vi "Periodic Tasks.vi"(8 "error in":errorcluster) -> ()   [LabVIEW 2019]
doc: "This VI runs in parallel to other tasks. It can contain as many user-defined periodic loops as you need. These can carry out PID or other sorts of timed response."
uses:
  <vilib>/Rock Robotics/WPI/Utilities/WPI_GetSetVariantRefNum.vi
  <vilib>/Rock Robotics/Network Tables/NT Read Boolean.vi
  <vilib>/Rock Robotics/Network Tables/NT Read Number.vi
  <vilib>/Rock Robotics/WPI/RobotDrive/WPI_RobotDriveArcadeDrive_Standard(NoSaturation).vi
  <vilib>/Rock Robotics/Network Tables/NT Write Numeric Array.vi
  <vilib>/Rock Robotics/Network Tables/NT Write Boolean.vi
  <vilib>/Rock Robotics/Network Tables/NT Write Number.vi
  <vilib>/Rock Robotics/Network Tables/NT Write String.vi
  <vilib>/Rock Robotics/Network Tables/NT Read String.vi
panel:
  out "Motor velocities":dbl[](array[knob]) scale=0.0..10.0
  out "Motor temperatures":dbl[](array[slide]) scale=100.0..250.0
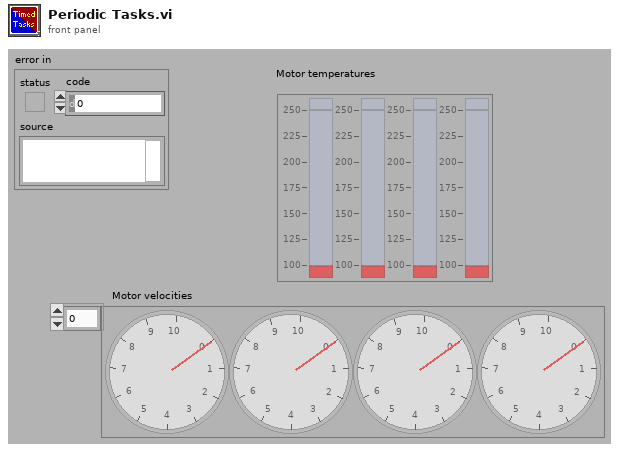
[diagram p1: front panel]
types:
  T1 = typedef "WPI_JoystickDevRef.ctl" = cluster{"Device":T2}
  T2 = typedef "WPI_JoystickDeviceEnum.ctl" = enum16{"USB 0", "USB 1", "USB 2", "USB 3", "USB 4", "USB 5"}
  T3 = typedef "WPI_RobotDriveDevRef.ctl" = cluster{"DevStatus":errorcluster, "Motors[]":T4[], "Square Inputs":bool, "Max Output":dbl}
  T4 = typedef "WPI_MotorControlDeviceRef.ctl" = cluster{"DeviceStatus":errorcluster, "Type":T5, "PWM":cluster{"PWM Channel":T6, "DeadBand":T7}, "CAN":cluster{"Device Number":u8, "SetOutput VI Ref":variant, "GetOutput VI Ref":variant, "Enable VI Ref":variant, "Disable VI Ref":variant, "Data":variant}, "Invert":bool, "DIO PWM":cluster{"PWM \"Enable\" Channel":T6, "DIOChannel":T8, "PWM Rate":dbl}}
  T5 = typedef "WPI_MotorControlType.ctl" = enum16{"PWM", "CAN", "DIO PWM"}
  T6 = typedef "FPGA_DIOPWMChannel.ctl" = enum8{"PWM 0", "PWM 1", "PWM 2", "PWM 3", "PWM 4", "PWM 5", "PWM 6", "PWM 7", "PWM 8", "PWM 9", "PWM MXP 0", "PWM MXP 1", "PWM MXP 2", "PWM MXP 3", "PWM MXP 4", "PWM MXP 5", "PWM MXP 6", "PWM MXP 7", "PWM MXP 8", "PWM MXP 9", "Invalid"}
  T7 = typedef "WPI_PWMDeadband.ctl" = cluster{"Name":string, "maxPositivePwm":i32, "minPositivePwm":i32, "centerPwm":i32, "maxNegativePwm":i32, "minNegativePwm":i32, "angularRange":u16}
  T8 = typedef "FPGA_DIOChannel.ctl" = enum8{"DIO 0", "DIO 1", "DIO 2", "DIO 3", "DIO 4", "DIO 5", "DIO 6", "DIO 7", "DIO 8", "DIO 9", "DIO MXP 0", "DIO MXP 1", "DIO MXP 2", "DIO MXP 3", "DIO MXP 4", "DIO MXP 5", "DIO MXP 6", "DIO MXP 7", "DIO MXP 8", "DIO MXP 9", "DIO MXP 10", "DIO MXP 11", "DIO MXP 12", "DIO MXP 13", "DIO MXP 14", "DIO MXP 15", "SPI Port CS1", "SPI Port CS2", "SPI Port CS3", "SPI Port MISO", "SPI Port MOSI", "Invalid"}
  T9 = cluster{"JoystickDevRef":T1, "RobotDriveDevRef":T3}
  T10 = typedef "Color Sensor V3 DevRef.ctl" = cluster{"I2CDevRef":T11}
  T11 = typedef "WPI_I2CDevRef.ctl" = cluster{"DevStatus":errorcluster, "Device Address":u8, "Handle":i32, "I2C Bus":T12}
  T12 = typedef "i2c_bus.ctl" = enum16{"I2C On-Board", "I2C MXP", "Invalid"}
  T13 = typedef "WPI_SwitchDevRef.ctl" = cluster{"DevStatus":errorcluster, "DIO Channel":T8, "CntIndex":T14, "Normally Closed":bool}
  T14 = typedef "FPGA_CounterCtrSystemIndex.ctl" = enum8{"Ctr 0", "Ctr 1", "Ctr 2", "Ctr 3", "Ctr 4", "Ctr 5", "Ctr 6", "Ctr 7", "Invalid"}
  T15 = typedef "WPI_ServoDeviceRef.ctl" = cluster{"DeviceStatus":errorcluster, "PWM Channel":T6, "DeadBand":T7}
  T16 = typedef "WPI_EncoderDevRef.ctl" = cluster{"DevStatus":errorcluster, "EncoderIndex":T17, "CounterIndex":T14, "DistancePerCount":dbl, "Decoding Type":T18}
  T17 = typedef "FPGA_EncoderIdx.ctl" = enum8{"Enc 0", "Enc 1", "Enc 2", "Enc 3", "Enc 4", "Enc 5", "Enc 6", "Enc 7", "Invalid"}
  T18 = typedef "WPI_EncoderType.ctl" = enum16{"1x", "2x", "4x"}
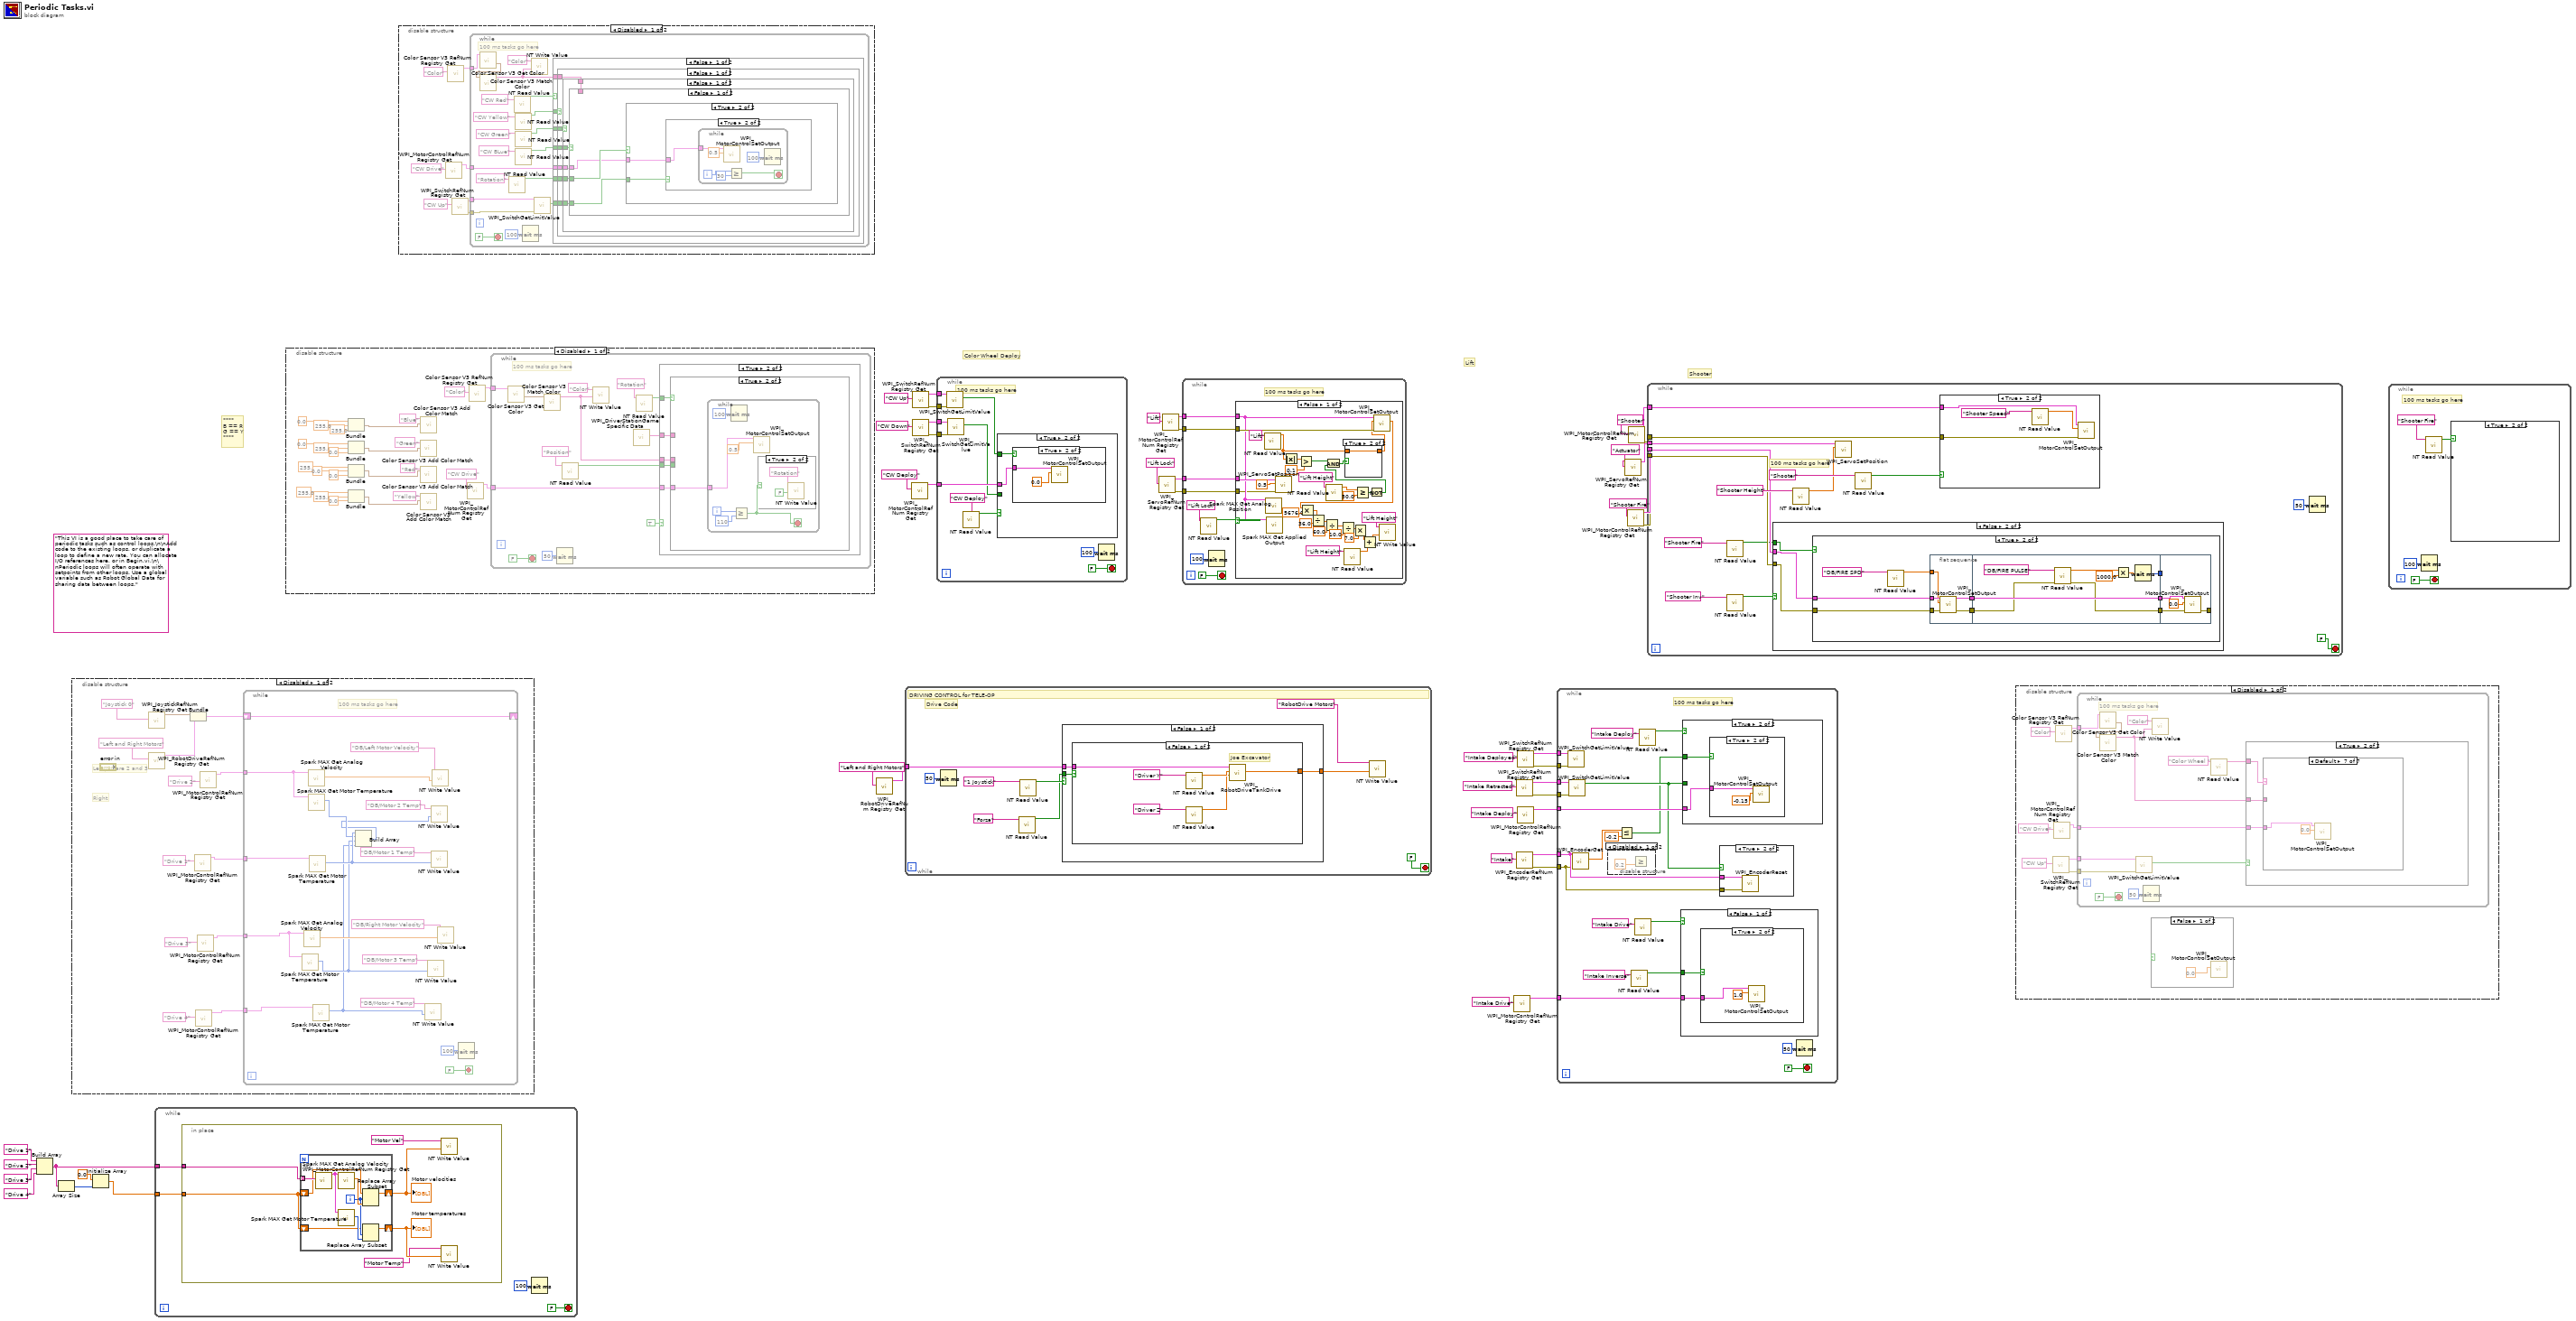
[diagram p0: block diagram]
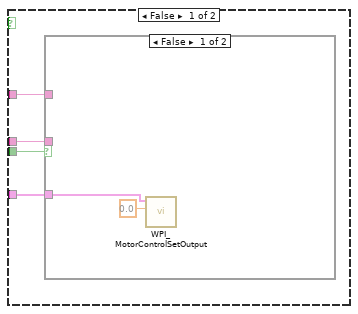
[diagram p3: hidden frame]
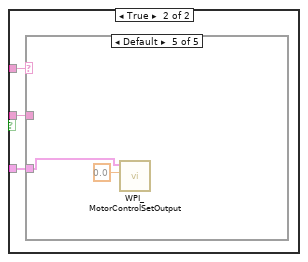
[diagram p4: hidden frame]
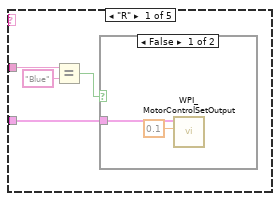
[diagram p5: hidden frame]
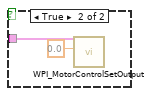
[diagram p6: hidden frame]
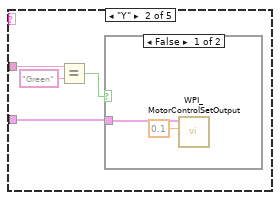
[diagram p7: hidden frame]
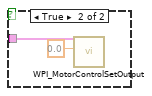
[diagram p8: hidden frame]
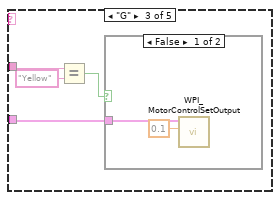
[diagram p9: hidden frame]
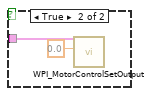
[diagram p10: hidden frame]
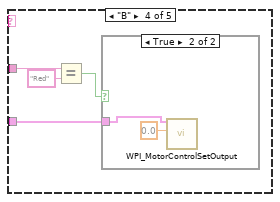
[diagram p11: hidden frame]
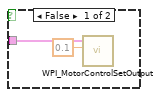
[diagram p12: hidden frame]
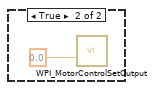
[diagram p16: hidden frame]
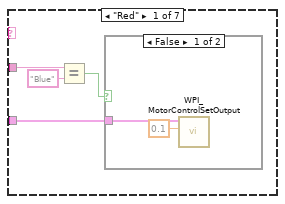
[diagram p18: hidden frame]
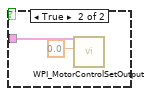
[diagram p19: hidden frame]
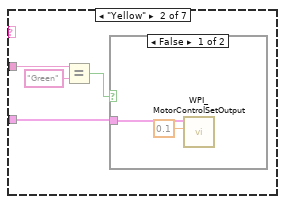
[diagram p20: hidden frame]
diagram:
  (unwired) "This VI is a good place to take care of periodic tasks such as control loops.\n\nAdd code to the existing loops, or duplicate a loop to define a new rate. You can allocate I/O references here, or in Begin.vi.\n\nPeriodic loops will often operate with setpoints from other loops. Use a global variable such as Robot Global Data for sharing data between loops."
  # "Shooter"
  # "Lift"
  # "****\nB == R\nG == Y\n****"
  # "Color Wheel Deploy"
  n1 = Build Array("Drive 1", "Drive 2", "Drive 3", "Drive 4") -> (w2:string[])
  n2 = Array Size(array=w2) -> (size(s)=w8:i32)
  n3 = disable-structure shown="Disabled" {
    frame Disabled {
      # "Right"
      # "Left"
      # "Masters are 2 and 3"
      n4 = call <vilib>:"WPI_JoystickRefNum Registry Get.vi"("refnum name"="Joystick 0") -> ("JoystickDevRef"=w56:T1)  [unwired: 1 in, 9 out]
      n5 = call <vilib>:"WPI_RobotDriveRefNum Registry Get.vi"("refnum name"="Left and Right Motors") -> ("RobotDriveDevRef"=w55:T3)  [unwired: 1 in, 9 out]
      n6 = Bundle("JoystickDevRef"=w56, "RobotDriveDevRef"=w55) -> (w54:T9)  [unwired: 1 out]
      n7 = call <vilib>:"WPI_MotorControlRefNum Registry Get.vi"("refnum name"="Drive 1") -> ("MotorControlDevRef"=w49:T4)  [unwired: 9 in, 1 out]
      n8 = call <vilib>:"WPI_MotorControlRefNum Registry Get.vi"("refnum name"="Drive 4") -> ("MotorControlDevRef"=w46:T4)  [unwired: 9 in, 1 out]
      n9 = call <vilib>:"WPI_MotorControlRefNum Registry Get.vi"("refnum name"="Drive 3") -> ("MotorControlDevRef"=w47:T4)  [unwired: 9 in, 1 out]
      n10 = call <vilib>:"WPI_MotorControlRefNum Registry Get.vi"("refnum name"="Drive 2") -> ("MotorControlDevRef"=w48:T4)  [unwired: 9 in, 1 out]
      n11 = while {
        shift-right: [w76] -> _
        shift-left: w54 -> [w76]
        tunnel: w49 -> [w60]
        tunnel: w48 -> [w69]
        tunnel: w47 -> [w68]
        tunnel: w46 -> [w67]
        stop <- FALSE stop-if-true
        # "100 ms tasks go here"
        n12 = call <vilib>:"Spark MAX Get Motor Temperature.vi"("MotorControlDevRef in"=w68) -> ("Motor Temperature"=w62:u8)  [unwired: 7 in, 3 out]
        n13 = call <vilib>:"Spark MAX Get Analog Velocity.vi"("MotorControlDevRef in"=w68) -> ("Analog Velocity"=w70:dbl)  [unwired: 7 in, 3 out]
        n14 = call <vilib>:"Spark MAX Get Analog Velocity.vi"("MotorControlDevRef in"=w69) -> ("Analog Velocity"=w73:dbl)  [unwired: 7 in, 3 out]
        n15 = call <vilib>:"Spark MAX Get Motor Temperature.vi"("MotorControlDevRef in"=w69) -> ("Motor Temperature"=w63:u8)  [unwired: 7 in, 3 out]
        n16 = call <vilib>:"Spark MAX Get Motor Temperature.vi"("MotorControlDevRef in"=w60) -> ("Motor Temperature"=w64:u8)  [unwired: 7 in, 3 out]
        n17 = call <vilib>:"Spark MAX Get Motor Temperature.vi"("MotorControlDevRef in"=w67) -> ("Motor Temperature"=w61:u8)  [unwired: 7 in, 3 out]
        n18 = Build Array(w64, w63, w62, w61) -> (w59:u8[])
        n19 = call-poly <vilib>:"NT Write Value.vi"("Numeric"=w61, "Name"="DB/Motor 4 Temp") -> ()  [unwired: 9 in, 1 out]
        n20 = call-poly <vilib>:"NT Write Value.vi"("Numeric"=w62, "Name"="DB/Motor 3 Temp") -> ()  [unwired: 9 in, 1 out]
        n21 = call-poly <vilib>:"NT Write Value.vi"("Numeric Array"=w59, "Name"="DB/Motor 2 Temp") -> ()  [unwired: 9 in, 1 out]
        n22 = call-poly <vilib>:"NT Write Value.vi"("Numeric"=w64, "Name"="DB/Motor 1 Temp") -> ()  [unwired: 9 in, 1 out]
        n23 = call-poly <vilib>:"NT Write Value.vi"("Numeric"=w73, "Name"="DB/Left Motor Velocity") -> ()  [unwired: 9 in, 1 out]
        n24 = call-poly <vilib>:"NT Write Value.vi"("Numeric"=w70, "Name"="DB/Right Motor Velocity") -> ()  [unwired: 9 in, 1 out]
        n25 = Wait (ms)(milliseconds to wait=u32 100) -> ()  [unwired: 1 out]
      }
    }
    frame Enabled {
    }
  }
  n26 = Initialize Array(0.0 ("element"), w8) -> (w1:dbl[])
  n27 = while {
    tunnel: w2 -> [w80]
    tunnel: w1 -> [w79]
    stop <- FALSE stop-if-true
    n28 = in-place {
      in-place-border: w80 -> [w84]
      in-place-border: w79 -> [w83]
      n29 = for {
        tunnel: w84 -> [w97] mode=indexing
        shift-right: [w92] -> w88
        shift-left: w83 -> [w89]
        shift-right: [w93] -> w86
        shift-left: w83 -> [w95]
        i -> [w91]
        n30 = call <vilib>:"WPI_MotorControlRefNum Registry Get.vi"("refnum name"=w97) -> ("MotorControlDevRef"=w96:T4)  [unwired: 9 in, 1 out]
        n31 = call <vilib>:"Spark MAX Get Analog Velocity.vi"("MotorControlDevRef in"=w96) -> ("Analog Velocity"=w94:dbl)  [unwired: 7 in, 3 out]
        n32 = call <vilib>:"Spark MAX Get Motor Temperature.vi"("MotorControlDevRef in"=w96) -> ("Motor Temperature"=w90:u8)  [unwired: 7 in, 3 out]
        n33 = Replace Array Subset(array=w95, new element=w94, index=w91) -> (w93:dbl[])
        n34 = Replace Array Subset(array=w89, new element=w90, index=w91) -> (w92:dbl[])
      }
      "Motor velocities" <- w86
      "Motor temperatures" <- w88
      n35 = call-poly <vilib>:"NT Write Value.vi"("Numeric Array"=w86, "Name"="Motor Vel") -> ()  [unwired: 9 in, 1 out]
      n36 = call-poly <vilib>:"NT Write Value.vi"("Numeric Array"=w88, "Name"="Motor Temp") -> ()  [unwired: 9 in, 1 out]
    }
    n37 = Wait (ms)(milliseconds to wait=u32 100) -> ()  [unwired: 1 out]
  }
  n38 = disable-structure shown="Disabled" {
    frame Disabled {
      n39 = Bundle(0.0, 255.0, 255.0) -> (w115:cluster{dbl, dbl, dbl})  [unwired: 1 in]
      n40 = Bundle(0.0, 255.0, 0.0) -> (w110:cluster{dbl, dbl, dbl})  [unwired: 1 in]
      n41 = Bundle(255.0, 0.0, 0.0) -> (w103:cluster{dbl, dbl, dbl})  [unwired: 1 in]
      n42 = Bundle(255.0, 255.0, 0.0) -> (w102:cluster{dbl, dbl, dbl})  [unwired: 1 in]
      n43 = call <vilib>:"Color Sensor V3 Add Color Match.vi"("Color"=w110, "Name"="Green") -> ()  [unwired: 10 in]
      n44 = call <vilib>:"Color Sensor V3 Add Color Match.vi"("Color"=w103, "Name"="Red") -> ()  [unwired: 10 in]
      n45 = call <vilib>:"Color Sensor V3 Add Color Match.vi"("Color"=w115, "Name"="Blue") -> ()  [unwired: 10 in]
      n46 = call <vilib>:"Color Sensor V3 Add Color Match.vi"("Color"=w102, "Name"="Yellow") -> ()  [unwired: 10 in]
      n47 = call <vilib>:"WPI_MotorControlRefNum Registry Get.vi"("refnum name"="CW Drive") -> ("MotorControlDevRef"=w98:T4)  [unwired: 9 in, 1 out]
      n48 = call <vilib>:"Color Sensor V3 RefNum Registry Get.vi"("refnum name"="Color") -> ("ColorSensorDevRef"=w100:T10)  [unwired: 9 in, 1 out]
      n49 = while {
        tunnel: w100 -> [w132]
        tunnel: w98 -> [w128]
        stop <- FALSE stop-if-true
        # "100 ms tasks go here"
        n50 = call <vilib>:"Color Sensor V3 Get Color.vi"("ColorSensorDevRef"=w132) -> ("Normalized Color"=w131:cluster{"R":dbl, "G":dbl, "B":dbl})  [unwired: 7 in, 3 out]
        n51 = call <vilib>:"Color Sensor V3 Match Color.vi"("Measured Color"=w131) -> ("Matched Color Name"=w129:string)  [unwired: 8 in, 2 out]
        n52 = Wait (ms)(milliseconds to wait=u32 50) -> ()  [unwired: 1 out]
        n53 = call-poly <vilib>:"NT Read Value.vi"("Name"="Position") -> ("Boolean"=w122:bool)  [unwired: 9 in, 1 out]
        n54 = call-poly <vilib>:"NT Write Value.vi"("String"=w129, "Name"="Color") -> ()  [unwired: 9 in, 1 out]
        n55 = call <vilib>:"WPI_DriverStationGame Specific Data.vi"() -> ("Game Specific Data"=w127:string)  [unwired: 11 in]
        n56 = call-poly <vilib>:"NT Read Value.vi"("Name"="Rotation") -> ("Boolean"=w125:bool)  [unwired: 9 in, 1 out]
        n57 = case shown="True" TRUE {
          tunnel: w127 -> [_ w138]
          tunnel: w129 -> [_ w137]
          tunnel: w128 -> [_ w136]
          tunnel: w125 -> [_ w139]
          tunnel: w122 -> [_ w135]
          frame False {
          }
          frame True {
            n58 = case shown="True" w139 {
              tunnel: w138 -> [w143 _]
              tunnel: w137 -> [w142 _]
              tunnel: w136 -> [w141 w183]
              tunnel: w135 -> [w140 _]
              frame False {
                n59 = case shown="False" w140 {
                  tunnel: w143 -> [_ w148]
                  tunnel: w142 -> [_ w147]
                  tunnel: w141 -> [w144 w146]
                  frame False {
                    n60 = call <vilib>:"WPI_MotorControlSetOutput.vi"("Output"=0.0, "MotorControlDevRef"=w144) -> ()  [unwired: 7 in, 3 out]
                  }
                  frame True {
                    n61 = case shown="Default" w148 {
                      tunnel: w147 -> [w152 w157 w166 w174 _]
                      tunnel: w146 -> [w150 w158 w165 w173 w181]
                      frame "R" {
                        n62 = Equal?(x=w152, y="Blue") -> (x = y?=w151:bool)
                        n63 = case shown="False" w151 {
                          tunnel: w150 -> [w154 w156]
                          frame False {
                            n64 = call <vilib>:"WPI_MotorControlSetOutput.vi"("Output"=0.1, "MotorControlDevRef"=w154) -> ()  [unwired: 7 in, 3 out]
                          }
                          frame True {
                            n65 = call <vilib>:"WPI_MotorControlSetOutput.vi"("Output"=0.0, "MotorControlDevRef"=w156) -> ()  [unwired: 7 in, 3 out]
                          }
                        }
                      }
                      frame "Y" {
                        n66 = Equal?(x=w157, y="Green") -> (x = y?=w160:bool)
                        n67 = case shown="False" w160 {
                          tunnel: w158 -> [w162 w164]
                          frame False {
                            n68 = call <vilib>:"WPI_MotorControlSetOutput.vi"("Output"=0.1, "MotorControlDevRef"=w162) -> ()  [unwired: 7 in, 3 out]
                          }
                          frame True {
                            n69 = call <vilib>:"WPI_MotorControlSetOutput.vi"("Output"=0.0, "MotorControlDevRef"=w164) -> ()  [unwired: 7 in, 3 out]
                          }
                        }
                      }
                      frame "G" {
                        n70 = Equal?(x=w166, y="Yellow") -> (x = y?=w168:bool)
                        n71 = case shown="False" w168 {
                          tunnel: w165 -> [w170 w172]
                          frame False {
                            n72 = call <vilib>:"WPI_MotorControlSetOutput.vi"("Output"=0.1, "MotorControlDevRef"=w170) -> ()  [unwired: 7 in, 3 out]
                          }
                          frame True {
                            n73 = call <vilib>:"WPI_MotorControlSetOutput.vi"("Output"=0.0, "MotorControlDevRef"=w172) -> ()  [unwired: 7 in, 3 out]
                          }
                        }
                      }
                      frame "B" {
                        n74 = Equal?(x=w174, y="Red") -> (x = y?=w176:bool)
                        n75 = case shown="True" w176 {
                          tunnel: w173 -> [w177 w179]
                          frame False {
                            n76 = call <vilib>:"WPI_MotorControlSetOutput.vi"("Output"=0.1, "MotorControlDevRef"=w177) -> ()  [unwired: 7 in, 3 out]
                          }
                          frame True {
                            n77 = call <vilib>:"WPI_MotorControlSetOutput.vi"("Output"=0.0, "MotorControlDevRef"=w179) -> ()  [unwired: 7 in, 3 out]
                          }
                        }
                      }
                      frame Default {
                        n78 = call <vilib>:"WPI_MotorControlSetOutput.vi"("Output"=0.0, "MotorControlDevRef"=w181) -> ()  [unwired: 7 in, 3 out]
                      }
                    }
                  }
                }
              }
              frame True {
                n79 = while {
                  tunnel: w183 -> [w184]
                  i -> [w188]
                  stop <- w186 stop-if-true
                  n80 = Wait (ms)(milliseconds to wait=u32 100) -> ()  [unwired: 1 out]
                  n81 = Greater Or Equal?(x=w188, y=110) -> (x >= y?=w186:bool)
                  n82 = call <vilib>:"WPI_MotorControlSetOutput.vi"("Output"=0.5, "MotorControlDevRef"=w184) -> ()  [unwired: 7 in, 3 out]
                  n83 = case shown="True" w186 {
                    frame False {
                    }
                    frame True {
                      n84 = call-poly <vilib>:"NT Write Value.vi"("Boolean"=FALSE, "Name"="Rotation") -> ()  [unwired: 9 in, 1 out]
                    }
                  }
                }
              }
            }
          }
        }
      }
    }
    frame Enabled {
    }
  }
  n85 = disable-structure shown="Disabled" {
    frame Disabled {
      n86 = call <vilib>:"WPI_MotorControlRefNum Registry Get.vi"("refnum name"="CW Drive") -> ("MotorControlDevRef"=w195:T4)  [unwired: 9 in, 1 out]
      n87 = call <vilib>:"Color Sensor V3 RefNum Registry Get.vi"("refnum name"="Color") -> ("ColorSensorDevRef"=w197:T10)  [unwired: 9 in, 1 out]
      n88 = call <vilib>:"WPI_SwitchRefNum Registry Get.vi"("refnum name"="CW Up") -> ("error out"=w192:errorcluster, "SwitchDevRef"=w193:T13)  [unwired: 9 in]
      n89 = while {
        tunnel: w197 -> [w216]
        tunnel: w195 -> [w206]
        tunnel: w193 -> [w203]
        tunnel: w192 -> [w202]
        stop <- FALSE stop-if-true
        # "100 ms tasks go here"
        n90 = call <vilib>:"Color Sensor V3 Get Color.vi"("ColorSensorDevRef"=w216) -> ("Normalized Color"=w215:cluster{"R":dbl, "G":dbl, "B":dbl})  [unwired: 7 in, 3 out]
        n91 = call <vilib>:"Color Sensor V3 Match Color.vi"("Measured Color"=w215) -> ("Matched Color Name"=w200:string)  [unwired: 8 in, 2 out]
        n92 = call-poly <vilib>:"NT Read Value.vi"("Name"="Rotation") -> ("Boolean"=w204:bool)  [unwired: 9 in, 1 out]
        n93 = call-poly <vilib>:"NT Read Value.vi"("Name"="CW Red") -> ("Boolean"=w211:bool)  [unwired: 9 in, 1 out]
        n94 = call-poly <vilib>:"NT Read Value.vi"("Name"="CW Yellow") -> ("Boolean"=w210:bool)  [unwired: 9 in, 1 out]
        n95 = call-poly <vilib>:"NT Read Value.vi"("Name"="CW BLue") -> ("Boolean"=w207:bool)  [unwired: 9 in, 1 out]
        n96 = call-poly <vilib>:"NT Read Value.vi"("Name"="CW Green") -> ("Boolean"=w209:bool)  [unwired: 9 in, 1 out]
        n97 = Wait (ms)(milliseconds to wait=u32 100) -> ()  [unwired: 1 out]
        n98 = call-poly <vilib>:"NT Write Value.vi"("String"=w200, "Name"="Color") -> ()  [unwired: 9 in, 1 out]
        n99 = call <vilib>:"WPI_SwitchGetLimitValue.vi"("error in (no error)"=w202, "SwitchDevRef"=w203) -> ("Switch Pressed"=w201:bool)  [unwired: 7 in, 2 out]
        n100 = case shown="False" w211 {
          tunnel: w210 -> [w225 _]
          tunnel: w209 -> [w224 _]
          tunnel: w207 -> [w223 _]
          tunnel: w200 -> [w222 w279]
          tunnel: w206 -> [w221 w277]
          tunnel: w204 -> [w220 _]
          tunnel: w201 -> [w219 _]
          frame False {
            n101 = case shown="False" w225 {
              tunnel: w224 -> [w231 _]
              tunnel: w223 -> [w230 _]
              tunnel: w222 -> [w229 w272]
              tunnel: w221 -> [w228 w269]
              tunnel: w220 -> [w227 _]
              tunnel: w219 -> [w226 _]
              frame False {
                n102 = case shown="False" w231 {
                  tunnel: w230 -> [w236 _]
                  tunnel: w229 -> [w235 w264]
                  tunnel: w228 -> [w234 w261]
                  tunnel: w227 -> [w233 _]
                  tunnel: w226 -> [w232 _]
                  frame False {
                    n103 = case shown="False" w236 {
                      tunnel: w235 -> [_ w254]
                      tunnel: w234 -> [w238 w253]
                      tunnel: w233 -> [w239 _]
                      tunnel: w232 -> [w237 _]
                      frame False {
                        n104 = case shown="True" w239 {
                          tunnel: w238 -> [w240 w243]
                          tunnel: w237 -> [_ w242]
                          frame False {
                            n105 = call <vilib>:"WPI_MotorControlSetOutput.vi"("Output"=0.0, "MotorControlDevRef"=w240) -> ()  [unwired: 7 in, 3 out]
                          }
                          frame True {
                            n106 = case shown="True" w242 {
                              tunnel: w243 -> [w244 w246]
                              frame False {
                                n107 = call <vilib>:"WPI_MotorControlSetOutput.vi"("Output"=0.0, "MotorControlDevRef"=w244) -> ()  [unwired: 7 in, 3 out]
                              }
                              frame True {
                                n108 = while {
                                tunnel: w246 -> [w251]
                                i -> [w249]
                                stop <- w247 stop-if-true
                                n109 = call <vilib>:"WPI_MotorControlSetOutput.vi"("Output"=0.5, "MotorControlDevRef"=w251) -> ()  [unwired: 7 in, 3 out]
                                n110 = Greater Or Equal?(x=w249, y=30) -> (x >= y?=w247:bool)
                                n111 = Wait (ms)(milliseconds to wait=u32 100) -> ()  [unwired: 1 out]
                                }
                              }
                            }
                          }
                        }
                      }
                      frame True {
                        n112 = Equal?(x=w254, y="Red") -> (x = y?=w255:bool)
                        n113 = case shown="False" w255 {
                          tunnel: w253 -> [w257 w259]
                          frame False {
                            n114 = call <vilib>:"WPI_MotorControlSetOutput.vi"("Output"=0.1, "MotorControlDevRef"=w257) -> ()  [unwired: 7 in, 3 out]
                          }
                          frame True {
                            n115 = call <vilib>:"WPI_MotorControlSetOutput.vi"("Output"=0.0, "MotorControlDevRef"=w259) -> ()  [unwired: 7 in, 3 out]
                          }
                        }
                      }
                    }
                  }
                  frame True {
                    n116 = Equal?(x=w264, y="Yellow") -> (x = y?=w262:bool)
                    n117 = case shown="True" w262 {
                      tunnel: w261 -> [w265 w267]
                      frame False {
                        n118 = call <vilib>:"WPI_MotorControlSetOutput.vi"("Output"=0.1, "MotorControlDevRef"=w265) -> ()  [unwired: 7 in, 3 out]
                      }
                      frame True {
                        n119 = call <vilib>:"WPI_MotorControlSetOutput.vi"("Output"=0.0, "MotorControlDevRef"=w267) -> ()  [unwired: 7 in, 3 out]
                      }
                    }
                  }
                }
              }
              frame True {
                n120 = Equal?(x=w272, y="Green") -> (x = y?=w271:bool)
                n121 = case shown="True" w271 {
                  tunnel: w269 -> [w273 w275]
                  frame False {
                    n122 = call <vilib>:"WPI_MotorControlSetOutput.vi"("Output"=0.1, "MotorControlDevRef"=w273) -> ()  [unwired: 7 in, 3 out]
                  }
                  frame True {
                    n123 = call <vilib>:"WPI_MotorControlSetOutput.vi"("Output"=0.0, "MotorControlDevRef"=w275) -> ()  [unwired: 7 in, 3 out]
                  }
                }
              }
            }
          }
          frame True {
            n124 = Equal?(x=w279, y="Blue") -> (x = y?=w280:bool)
            n125 = case shown="True" w280 {
              tunnel: w277 -> [w281 w283]
              frame False {
                n126 = call <vilib>:"WPI_MotorControlSetOutput.vi"("Output"=0.1, "MotorControlDevRef"=w281) -> ()  [unwired: 7 in, 3 out]
              }
              frame True {
                n127 = call <vilib>:"WPI_MotorControlSetOutput.vi"("Output"=0.0, "MotorControlDevRef"=w283) -> ()  [unwired: 7 in, 3 out]
              }
            }
          }
        }
      }
    }
    frame Enabled {
    }
  }
  n128 = call <vilib>:"WPI_RobotDriveRefNum Registry Get.vi"("refnum name"="Left and Right Motors") -> ("RobotDriveDevRef"=w45:T3)  [unwired: 9 in, 1 out]
  n129 = while {
    tunnel: w45 -> [w291]
    stop <- FALSE stop-if-true
    # "Drive Code"
    # "DRIVING CONTROL for TELE-OP"
    n130 = Wait (ms)(milliseconds to wait=u32 50) -> ()  [unwired: 1 out]
    n131 = call-poly <vilib>:"NT Read Value.vi"("Name"="Forza") -> ("Boolean"=w285:bool)  [unwired: 9 in, 1 out]
    n132 = call-poly <vilib>:"NT Read Value.vi"("Name"="1 Joystick") -> ("Boolean"=w289:bool)  [unwired: 9 in, 1 out]
    n133 = case shown="False" w289 {
      tunnel: w291 -> [w296 w310]
      tunnel: [w295 w309] -> w288
      tunnel: w285 -> [w294 _]
      frame False {
        n134 = case shown="False" w294 {
          tunnel: w296 -> [w297 w304]
          tunnel: [w300 w303] -> w295
          frame False {
            # "Joe Excavator"
            n135 = call-poly <vilib>:"NT Read Value.vi"("Name"="Driver Y") -> ("Numeric"=w299:dbl)  [unwired: 9 in, 1 out]
            n136 = call-poly <vilib>:"NT Read Value.vi"("Name"="Driver Z") -> ("Numeric"=w298:dbl)  [unwired: 9 in, 1 out]
            n137 = call <vilib>:"WPI_RobotDriveTankDrive.vi"("Right axis value"=w298, "Left axis value"=w299, "RobotDriveDevRef"=w297) -> ("Motor Values"=w300:dbl[])  [unwired: 6 in, 2 out]
          }
          frame True {
            # "Nathan Forza"
            n138 = call-poly <vilib>:"NT Read Value.vi"("Name"="Driver Y") -> ("Numeric"=w306:dbl)  [unwired: 9 in, 1 out]
            n139 = call-poly <vilib>:"NT Read Value.vi"("Name"="Driver Z") -> ("Numeric"=w305:dbl)  [unwired: 9 in, 1 out]
            n140 = call-poly <vilib>:"WPI_RobotDriveArcadeDrive.vi"("Y axis value"=w305, "X axis value"=w306, "RobotDriveDevRef"=w304) -> ("Motor Values"=w303:dbl[])  [unwired: 6 in, 2 out]
          }
        }
      }
      frame True {
        # "\"1 Joystick\" = TRUE"
        n141 = in-place {
          in-place-border: [w314] -> w312
          in-place-border: [w313] -> w311
          # "twist-to-turn"
          n142 = call-poly <vilib>:"NT Read Value.vi"("Name"="Driver Y") -> ("Numeric"=w314:dbl)  [unwired: 9 in, 1 out]
          n143 = call-poly <vilib>:"NT Read Value.vi"("Name"="Driver Z") -> ("Numeric"=w313:dbl)  [unwired: 9 in, 1 out]
        }
        n144 = call-poly <vilib>:"WPI_RobotDriveArcadeDrive.vi"("Y axis value"=w311, "X axis value"=w312, "RobotDriveDevRef"=w310) -> ("Motor Values"=w309:dbl[])  [unwired: 6 in, 2 out]
      }
    }
    n145 = call-poly <vilib>:"NT Write Value.vi"("Numeric Array"=w288, "Name"="RobotDrive Motors") -> ()  [unwired: 9 in, 1 out]
  }
  n146 = call <vilib>:"WPI_MotorControlRefNum Registry Get.vi"("refnum name"="CW Deploy") -> ("MotorControlDevRef"=w36:T4)  [unwired: 9 in, 1 out]
  n147 = call <vilib>:"WPI_SwitchRefNum Registry Get.vi"("refnum name"="CW Up") -> ("error out"=w14:errorcluster, "SwitchDevRef"=w13:T13)  [unwired: 9 in]
  n148 = call <vilib>:"WPI_SwitchRefNum Registry Get.vi"("refnum name"="CW Down") -> ("error out"=w16:errorcluster, "SwitchDevRef"=w15:T13)  [unwired: 9 in]
  n149 = while {
    tunnel: w36 -> [w323]
    tunnel: w16 -> [w322]
    tunnel: w15 -> [w321]
    tunnel: w14 -> [w319]
    tunnel: w13 -> [w318]
    stop <- FALSE stop-if-true
    # "100 ms tasks go here"
    n150 = call <vilib>:"WPI_SwitchGetLimitValue.vi"("error in (no error)"=w319, "SwitchDevRef"=w318) -> ("Switch Pressed"=w317:bool)  [unwired: 7 in, 2 out]
    n151 = call <vilib>:"WPI_SwitchGetLimitValue.vi"("error in (no error)"=w322, "SwitchDevRef"=w321) -> ("Switch Pressed"=w320:bool)  [unwired: 7 in, 2 out]
    n152 = call-poly <vilib>:"NT Read Value.vi"("Name"="CW Deploy") -> ("Boolean"=w324:bool)  [unwired: 9 in, 1 out]
    n153 = case shown="True" w324 {
      tunnel: w323 -> [w329 w334]
      tunnel: w320 -> [w328 _]
      tunnel: w317 -> [_ w335]
      frame False {
        n154 = case shown="False" w328 {
          tunnel: w329 -> [w330 w333]
          frame False {
            n155 = call <vilib>:"WPI_MotorControlSetOutput.vi"("Output"=-0.2 ("Motor Output"), "MotorControlDevRef"=w330) -> ()  [unwired: 7 in, 3 out]
          }
          frame True {
            n156 = call <vilib>:"WPI_MotorControlSetOutput.vi"("Output"=0.0 ("Motor Output"), "MotorControlDevRef"=w333) -> ()  [unwired: 7 in, 3 out]
          }
        }
      }
      frame True {
        n157 = case shown="True" w335 {
          tunnel: w334 -> [w336 w339]
          frame False {
            n158 = call <vilib>:"WPI_MotorControlSetOutput.vi"("Output"=0.4 ("Motor Output"), "MotorControlDevRef"=w336) -> ()  [unwired: 7 in, 3 out]
          }
          frame True {
            n159 = call <vilib>:"WPI_MotorControlSetOutput.vi"("Output"=0.0 ("Motor Output"), "MotorControlDevRef"=w339) -> ()  [unwired: 7 in, 3 out]
          }
        }
      }
    }
    n160 = Wait (ms)(milliseconds to wait=u32 100) -> ()  [unwired: 1 out]
  }
  n161 = call <vilib>:"WPI_ServoRefNum Registry Get.vi"("refnum name"="Lift Lock") -> ("error out"=w12:errorcluster, "ServoDeviceRef"=w23:T15)  [unwired: 9 in]
  n162 = call <vilib>:"WPI_MotorControlRefNum Registry Get.vi"("refnum name"="Lift") -> ("error out"=w30:errorcluster, "MotorControlDevRef"=w31:T4)  [unwired: 9 in]
  n163 = while {
    tunnel: w31 -> [w340]
    tunnel: w30 -> [w341]
    tunnel: w23 -> [w345]
    tunnel: w12 -> [w342]
    stop <- FALSE stop-if-true
    # "100 ms tasks go here"
    n164 = call-poly <vilib>:"NT Read Value.vi"("Name"="Lift Lock") -> ("Boolean"=w343:bool)  [unwired: 9 in, 1 out]
    n165 = Wait (ms)(milliseconds to wait=u32 100) -> ()  [unwired: 1 out]
    n166 = case shown="False" w343 {
      tunnel: w345 -> [w379 w387]
      tunnel: w342 -> [w368 w386]
      tunnel: w341 -> [w377 w383]
      tunnel: w340 -> [w371 w384]
      frame False {
        n167 = call-poly <vilib>:"NT Read Value.vi"("Name"="Lift") -> ("Numeric"=w372:dbl)  [unwired: 9 in, 1 out]
        n168 = call <vilib>:"Spark MAX Get Analog Position.vi"("MotorControlDevRef in"=w371) -> ()  [unwired: 7 in, 4 out]
        n169 = call <vilib>:"Spark MAX Get Applied Output.vi"("MotorControlDevRef in"=w371) -> ()  [unwired: 7 in, 4 out]
        n170 = call <vilib>:"WPI_ServoSetPosition.vi"("error in (no error)"=w368, "Position"=0.5, "ServoDeviceRef"=w379) -> ()  [unwired: 7 in, 2 out]
        n171 = Absolute Value(x=w372) -> (abs(x)=w375:dbl)
        n172 = Greater?(x=w375, y=0.1) -> (0:w351:bool)
        n173 = call-poly <vilib>:"NT Read Value.vi"("Name"="Lift Height") -> ("Numeric"=w353:dbl)  [unwired: 9 in, 1 out]
        n174 = call-poly <vilib>:"NT Read Value.vi"("Name"="Lift Height") -> ("Numeric"=w356:dbl)  [unwired: 9 in, 1 out]
        n175 = Greater Or Equal?(x=w353, y=50.0) -> (x >= y?=w349:bool)
        n176 = Not(x=w349) -> (.not. x?=w348:bool)
        n177 = And(x=w351, y=w348) -> (x .and. y?=w350:bool)
        n178 = case shown="True" w350 {
          tunnel: [0.0 w381] -> w373
          tunnel: w372 -> [_ w381]
          frame False {
          }
          frame True {
          }
        }
        n179 = call <vilib>:"WPI_MotorControlSetOutput.vi"("error in (no error)"=w377, "Output"=w373, "MotorControlDevRef"=w371) -> ("Motor Output"=w360:dbl)  [unwired: 6 in, 2 out]
        n180 = Multiply(x=w360, y=5676.0) -> (x*y=w362:dbl)
        n181 = Divide(x=w362, y=36.0) -> (x/y=w365:dbl)
        n182 = Divide(x=w365, y=60.0) -> (x/y=w366:dbl)
        n183 = Divide(x=w366, y=10.0) -> (x/y=w364:dbl)
        n184 = Multiply(x=w364, y=7.0) -> (x*y=w355:dbl)
        n185 = Add(x=w355, y=w356) -> (x+y=w357:dbl)
        n186 = call-poly <vilib>:"NT Write Value.vi"("Numeric"=w357, "Name"="Lift Height") -> ()  [unwired: 9 in, 1 out]
      }
      frame True {
        n187 = call <vilib>:"WPI_ServoSetPosition.vi"("error in (no error)"=w386, "Position"=0.0, "ServoDeviceRef"=w387) -> ()  [unwired: 7 in, 2 out]
        n188 = call <vilib>:"WPI_MotorControlSetOutput.vi"("error in (no error)"=w383, "Output"=0.0, "MotorControlDevRef"=w384) -> ()  [unwired: 6 in, 3 out]
      }
    }
  }
  n189 = call <vilib>:"WPI_MotorControlRefNum Registry Get.vi"("refnum name"="Intake Drive") -> ("MotorControlDevRef"=w40:T4)  [unwired: 9 in, 1 out]
  n190 = call <vilib>:"WPI_SwitchRefNum Registry Get.vi"("refnum name"="Intake Retracted") -> ("error out"=w17:errorcluster, "SwitchDevRef"=w18:T13)  [unwired: 9 in]
  n191 = call <vilib>:"WPI_EncoderRefNum Registry Get.vi"("refnum name"="Intake") -> ("error out"=w11:errorcluster, "EncoderDevRef"=w10:T16)  [unwired: 9 in]
  n192 = call <vilib>:"WPI_SwitchRefNum Registry Get.vi"("refnum name"="Intake Deployed") -> ("error out"=w21:errorcluster, "SwitchDevRef"=w22:T13)  [unwired: 9 in]
  n193 = call <vilib>:"WPI_MotorControlRefNum Registry Get.vi"("refnum name"="Intake Deploy") -> ("MotorControlDevRef"=w42:T4)  [unwired: 9 in, 1 out]
  n194 = while {
    tunnel: w42 -> [w403]
    tunnel: w40 -> [w400]
    tunnel: w22 -> [w397]
    tunnel: w21 -> [w396]
    tunnel: w18 -> [w395]
    tunnel: w17 -> [w394]
    tunnel: w11 -> [w391]
    tunnel: w10 -> [w392]
    stop <- FALSE stop-if-true
    # "100 ms tasks go here"
    n195 = call <vilib>:"WPI_SwitchGetLimitValue.vi"("error in (no error)"=w396, "SwitchDevRef"=w397) -> ()  [unwired: 7 in, 3 out]
    n196 = call <vilib>:"WPI_SwitchGetLimitValue.vi"("error in (no error)"=w394, "SwitchDevRef"=w395) -> ("Switch Pressed"=w393:bool)  [unwired: 7 in, 2 out]
    n197 = call <vilib>:"WPI_EncoderGet.vi"("error in (no error)"=w391, "EncoderDevRef"=w392) -> ("Distance"=w388:dbl)  [unwired: 4 in, 5 out]
    n198 = disable-structure shown="Disabled" {
      frame Disabled {
        n199 = Greater Or Equal?(y=0.2) -> ()  [unwired: 1 in, 1 out]
      }
      frame Enabled {
      }
    }
    n200 = Less Or Equal?(x=w388, y=-0.2) -> (x <= y?=w389:bool)
    n201 = call-poly <vilib>:"NT Read Value.vi"("Name"="Intake Inverse") -> ("Boolean"=w398:bool)  [unwired: 9 in, 1 out]
    n202 = call-poly <vilib>:"NT Read Value.vi"("Name"="Intake Drive") -> ("Boolean"=w402:bool)  [unwired: 9 in, 1 out]
    n203 = call-poly <vilib>:"NT Read Value.vi"("Name"="Intake Deploy") -> ("Boolean"=w405:bool)  [unwired: 9 in, 1 out]
    n204 = case shown="False" w402 {
      tunnel: w400 -> [w411 w417]
      tunnel: w398 -> [w412 _]
      frame False {
        n205 = case shown="True" w412 {
          tunnel: w411 -> [w413 w415]
          frame False {
            n206 = call <vilib>:"WPI_MotorControlSetOutput.vi"("Output"=0.0, "MotorControlDevRef"=w413) -> ()  [unwired: 7 in, 3 out]
          }
          frame True {
            n207 = call <vilib>:"WPI_MotorControlSetOutput.vi"("Output"=1.0, "MotorControlDevRef"=w415) -> ()  [unwired: 7 in, 3 out]
          }
        }
      }
      frame True {
        n208 = call <vilib>:"WPI_MotorControlSetOutput.vi"("Output"=-1.0, "MotorControlDevRef"=w417) -> ()  [unwired: 7 in, 3 out]
      }
    }
    n209 = case shown="True" w405 {
      tunnel: w403 -> [w419 w422]
      tunnel: w393 -> [_ _]
      tunnel: w389 -> [_ w421]
      frame False {
        n210 = call <vilib>:"WPI_MotorControlSetOutput.vi"("Output"=0.0, "MotorControlDevRef"=w419) -> ()  [unwired: 7 in, 3 out]
      }
      frame True {
        n211 = case shown="True" w421 {
          tunnel: w422 -> [w423 w425]
          frame False {
            n212 = call <vilib>:"WPI_MotorControlSetOutput.vi"("Output"=-1.0, "MotorControlDevRef"=w423) -> ()  [unwired: 7 in, 3 out]
          }
          frame True {
            n213 = call <vilib>:"WPI_MotorControlSetOutput.vi"("Output"=-0.15, "MotorControlDevRef"=w425) -> ()  [unwired: 7 in, 3 out]
          }
        }
      }
    }
    n214 = case shown="True" w393 {
      tunnel: w392 -> [_ w410]
      tunnel: w391 -> [_ w409]
      frame False {
      }
      frame True {
        n215 = call <vilib>:"WPI_EncoderReset.vi"("error in (no error)"=w409, "EncoderDevRef"=w410) -> ()  [unwired: 8 in, 2 out]
      }
    }
    n216 = Wait (ms)(milliseconds to wait=u32 50) -> ()  [unwired: 1 out]
  }
  n217 = call <vilib>:"WPI_ServoRefNum Registry Get.vi"("refnum name"="Actuator") -> ("ServoDeviceRef"=w25:T15)  [unwired: 9 in, 1 out]
  n218 = call <vilib>:"WPI_MotorControlRefNum Registry Get.vi"("refnum name"="Shooter Fire") -> ("error out"=w27:errorcluster, "MotorControlDevRef"=w28:T4)  [unwired: 9 in]
  n219 = call <vilib>:"WPI_MotorControlRefNum Registry Get.vi"("refnum name"="Shooter") -> ("error out"=w33:errorcluster, "MotorControlDevRef"=w34:T4)  [unwired: 9 in]
  n220 = while {
    tunnel: w34 -> [w437]
    tunnel: w33 -> [w436]
    tunnel: w28 -> [w431]
    tunnel: w27 -> [w430]
    tunnel: w25 -> [w434]
    stop <- FALSE stop-if-true
    # "100 ms tasks go here"
    n221 = call-poly <vilib>:"NT Read Value.vi"("Name"="Shooter Fire") -> ("Boolean"=w429:bool)  [unwired: 9 in, 1 out]
    n222 = call-poly <vilib>:"NT Read Value.vi"("Name"="Shooter Inv") -> ("Boolean"=w427:bool)  [unwired: 9 in, 1 out]
    n223 = case shown="False" w427 {
      tunnel: w431 -> [w443 w458]
      tunnel: w430 -> [w442 w457]
      tunnel: w429 -> [_ w456]
      frame True {
        n224 = while {
          tunnel: w443 -> [w447]
          tunnel: w442 -> [w446]
          i -> [w452]
          stop <- w449 stop-if-true
          n225 = call <vilib>:"WPI_MotorControlSetOutput.vi"("error in (no error)"=w446, "Output"=-0.2, "MotorControlDevRef"=w447) -> ()  [unwired: 6 in, 3 out]
          n226 = Greater?(x=2, y=3) -> (0:w448:bool)
          n227 = Greater?(x=w452, y=4) -> (0:w449:bool)
          n228 = case shown="True" w448 {
            frame False {
            }
            frame True {
              n229 = call-poly <vilib>:"NT Write Value.vi"("Boolean"=FALSE, "Name"="Shooter Inv") -> ()  [unwired: 9 in, 1 out]
            }
          }
          n230 = Wait (ms)(milliseconds to wait=u32 50) -> ()  [unwired: 1 out]
        }
      }
      frame False {
        n231 = case shown="True" w456 {
          tunnel: w458 -> [w460 w470]
          tunnel: w457 -> [w459 w469]
          frame False {
            n232 = call <vilib>:"WPI_MotorControlSetOutput.vi"("error in (no error)"=w459, "Output"=0.0, "MotorControlDevRef"=w460) -> ()  [unwired: 6 in, 3 out]
          }
          frame True {
            n233 = call-poly <vilib>:"NT Read Value.vi"("Name"="DB/FIRE SPD") -> ("Numeric"=w467:dbl)  [unwired: 9 in, 1 out]
            n234 = flat-sequence {
              tunnel: w470 -> [w475]
              tunnel: w469 -> [w474]
              tunnel: w467 -> [w473]
              tunnel: [w472] -> w465
              tunnel: [w471] -> w464
              tunnel: [w483] -> w466
              tunnel: w465 -> [w483]
              tunnel: w464 -> [w478]
              tunnel: [w477] -> w463
              tunnel: [w476] -> w462
              tunnel: w466 -> [w487]
              tunnel: [w486] -> _
              tunnel: w463 -> [w485]
              tunnel: w462 -> [_]
              frame #0 {
                n235 = call <vilib>:"WPI_MotorControlSetOutput.vi"("error in (no error)"=w474, "Output"=w473, "MotorControlDevRef"=w475) -> ("error out"=w471:errorcluster, "MotorControlDevRef"=w472:T4)  [unwired: 6 in, 1 out]
              }
              frame #1 {
                n236 = call-poly <vilib>:"NT Read Value.vi"("error in"=w478, "Name"="DB/FIRE PULSE") -> ("error out"=w477:errorcluster, "Numeric"=w482:dbl)  [unwired: 8 in]
                n237 = Multiply(x=w482, y=1000.0) -> (x*y=w480:dbl)
                n238 = Wait (ms)(milliseconds to wait=w480) -> (millisecond timer value=w476:u32)
              }
              frame #2 {
                n239 = call <vilib>:"WPI_MotorControlSetOutput.vi"("error in (no error)"=w485, "Output"=0.0, "MotorControlDevRef"=w487) -> ("error out"=w486:errorcluster)  [unwired: 6 in, 2 out]
              }
            }
          }
        }
      }
    }
    n240 = call-poly <vilib>:"NT Read Value.vi"("Name"="Shooter Height") -> ("Numeric"=w432:dbl)  [unwired: 9 in, 1 out]
    n241 = call <vilib>:"WPI_ServoSetPosition.vi"("Position"=w432, "ServoDeviceRef"=w434) -> ()  [unwired: 8 in, 2 out]
    n242 = call-poly <vilib>:"NT Read Value.vi"("Name"="Shooter") -> ("Boolean"=w438:bool)  [unwired: 9 in, 1 out]
    n243 = case shown="True" w438 {
      tunnel: w437 -> [w489 w494]
      tunnel: w436 -> [w488 w493]
      frame False {
        n244 = call <vilib>:"WPI_MotorControlSetOutput.vi"("error in (no error)"=w488, "Output"=0.0, "MotorControlDevRef"=w489) -> ()  [unwired: 6 in, 3 out]
      }
      frame True {
        n245 = call-poly <vilib>:"NT Read Value.vi"("Name"="Shooter Speed") -> ("Numeric"=w491:dbl)  [unwired: 9 in, 1 out]
        n246 = call <vilib>:"WPI_MotorControlSetOutput.vi"("error in (no error)"=w493, "Output"=w491, "MotorControlDevRef"=w494) -> ()  [unwired: 6 in, 3 out]
      }
    }
    n247 = Wait (ms)(milliseconds to wait=u32 50) -> ()  [unwired: 1 out]
  }
  n248 = disable-structure shown="Disabled" {
    frame Disabled {
      n249 = call <vilib>:"WPI_SwitchRefNum Registry Get.vi"("refnum name"="CW Up") -> ("error out"=w495:errorcluster, "SwitchDevRef"=w496:T13)  [unwired: 9 in]
      n250 = call <vilib>:"WPI_MotorControlRefNum Registry Get.vi"("refnum name"="CW Drive") -> ("MotorControlDevRef"=w498:T4)  [unwired: 9 in, 1 out]
      n251 = call <vilib>:"Color Sensor V3 RefNum Registry Get.vi"("refnum name"="Color") -> ("ColorSensorDevRef"=w500:T10)  [unwired: 9 in, 1 out]
      n252 = while {
        tunnel: w500 -> [w513]
        tunnel: w498 -> [w504]
        tunnel: w496 -> [w511]
        tunnel: w495 -> [w510]
        stop <- FALSE stop-if-true
        # "100 ms tasks go here"
        n253 = call <vilib>:"Color Sensor V3 Get Color.vi"("ColorSensorDevRef"=w513) -> ("Normalized Color"=w512:cluster{"R":dbl, "G":dbl, "B":dbl})  [unwired: 7 in, 3 out]
        n254 = call <vilib>:"Color Sensor V3 Match Color.vi"("Measured Color"=w512) -> ("Matched Color Name"=w505:string)  [unwired: 8 in, 2 out]
        n255 = call <vilib>:"WPI_SwitchGetLimitValue.vi"("error in (no error)"=w510, "SwitchDevRef"=w511) -> ("Switch Pressed"=w507:bool)  [unwired: 7 in, 2 out]
        n256 = Wait (ms)(milliseconds to wait=u32 50) -> ()  [unwired: 1 out]
        n257 = call-poly <vilib>:"NT Write Value.vi"("String"=w505, "Name"="Color") -> ()  [unwired: 9 in, 1 out]
        n258 = call-poly <vilib>:"NT Read Value.vi"("Name"="Color Wheel ") -> ("String"=w506:string)  [unwired: 9 in, 1 out]
        n259 = case shown="True" w507 {
          tunnel: w506 -> [_ w518]
          tunnel: w505 -> [_ w517]
          tunnel: w504 -> [_ w516]
          frame False {
          }
          frame True {
            n260 = case shown="Default" w518 {
              tunnel: w517 -> [w522 w527 w536 w544 _ _ _]
              tunnel: w516 -> [w520 w528 w535 w543 w551 w554 w555]
              frame "Red" {
                n261 = Equal?(x=w522, y="Blue") -> (x = y?=w521:bool)
                n262 = case shown="False" w521 {
                  tunnel: w520 -> [w524 w526]
                  frame False {
                    n263 = call <vilib>:"WPI_MotorControlSetOutput.vi"("Output"=0.1, "MotorControlDevRef"=w524) -> ()  [unwired: 7 in, 3 out]
                  }
                  frame True {
                    n264 = call <vilib>:"WPI_MotorControlSetOutput.vi"("Output"=0.0, "MotorControlDevRef"=w526) -> ()  [unwired: 7 in, 3 out]
                  }
                }
              }
              frame "Yellow" {
                n265 = Equal?(x=w527, y="Green") -> (x = y?=w530:bool)
                n266 = case shown="False" w530 {
                  tunnel: w528 -> [w532 w534]
                  frame False {
                    n267 = call <vilib>:"WPI_MotorControlSetOutput.vi"("Output"=0.1, "MotorControlDevRef"=w532) -> ()  [unwired: 7 in, 3 out]
                  }
                  frame True {
                    n268 = call <vilib>:"WPI_MotorControlSetOutput.vi"("Output"=0.0, "MotorControlDevRef"=w534) -> ()  [unwired: 7 in, 3 out]
                  }
                }
              }
              frame "Green" {
                n269 = Equal?(x=w536, y="Yellow") -> (x = y?=w538:bool)
                n270 = case shown="False" w538 {
                  tunnel: w535 -> [w540 w542]
                  frame False {
                    n271 = call <vilib>:"WPI_MotorControlSetOutput.vi"("Output"=0.1, "MotorControlDevRef"=w540) -> ()  [unwired: 7 in, 3 out]
                  }
                  frame True {
                    n272 = call <vilib>:"WPI_MotorControlSetOutput.vi"("Output"=0.0, "MotorControlDevRef"=w542) -> ()  [unwired: 7 in, 3 out]
                  }
                }
              }
              frame "Blue" {
                n273 = Equal?(x=w544, y="Red") -> (x = y?=w546:bool)
                n274 = case shown="True" w546 {
                  tunnel: w543 -> [w547 w549]
                  frame False {
                    n275 = call <vilib>:"WPI_MotorControlSetOutput.vi"("Output"=0.1, "MotorControlDevRef"=w547) -> ()  [unwired: 7 in, 3 out]
                  }
                  frame True {
                    n276 = call <vilib>:"WPI_MotorControlSetOutput.vi"("Output"=0.0, "MotorControlDevRef"=w549) -> ()  [unwired: 7 in, 3 out]
                  }
                }
              }
              frame "Rotation" {
                n277 = call <vilib>:"WPI_MotorControlSetOutput.vi"("Output"=0.2, "MotorControlDevRef"=w551) -> ()  [unwired: 7 in, 3 out]
              }
              frame "Off" {
                n278 = call <vilib>:"WPI_MotorControlSetOutput.vi"("Output"=0.0, "MotorControlDevRef"=w554) -> ()  [unwired: 7 in, 3 out]
              }
              frame Default {
                n279 = call <vilib>:"WPI_MotorControlSetOutput.vi"("Output"=0.0, "MotorControlDevRef"=w555) -> ()  [unwired: 7 in, 3 out]
              }
            }
          }
        }
      }
      n280 = case shown="False" {
        selector: _ -> [_ _]
        frame False {
          n281 = call <vilib>:"WPI_MotorControlSetOutput.vi"("Output"=0.0) -> ()  [unwired: 8 in, 3 out]
        }
        frame True {
          n282 = call <vilib>:"WPI_MotorControlSetOutput.vi"("Output"=0.0) -> ()  [unwired: 8 in, 3 out]
        }
      }
    }
    frame Enabled {
    }
  }
  n283 = while {
    stop <- FALSE stop-if-true
    # "100 ms tasks go here"
    n284 = Wait (ms)(milliseconds to wait=u32 100) -> ()  [unwired: 1 out]
    n285 = call-poly <vilib>:"NT Read Value.vi"("Name"="Shooter Fire") -> ("Boolean"=w557:bool)  [unwired: 9 in, 1 out]
    n286 = case shown="True" w557 {
      frame False {
      }
      frame True {
      }
    }
  }
